vi "dialog.query_string_lua.vi"(5 "LuaVIEW reference":T1) -> (15 "error out":errorcluster)   [LabVIEW 2012]
doc: "Queries for a string by means of a dialog with a string control and OK/Cancel buttons.\nParameters:\nstr:prompt, prompt to display in the dialog titel bar.\n[str:default], default string to set the string control to.\nResults:\nbool:ok, set to true when the query was OKed, false when cancelled.\nstr:string, the entered string."
uses:
  typedefs/t_LuaVIEW Reference.ctl
  subvis/private/LuaVIEW Pull (string).vi
  subvis/private/LuaVIEW Push (boolean).vi
  subvis/private/LuaVIEW Push (string).vi
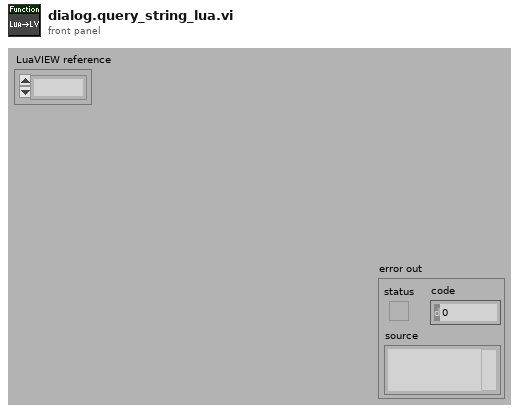
[diagram p1: front panel]
types:
  T1 = typedef "t_LuaVIEW Reference.ctl" = refnum<k1>
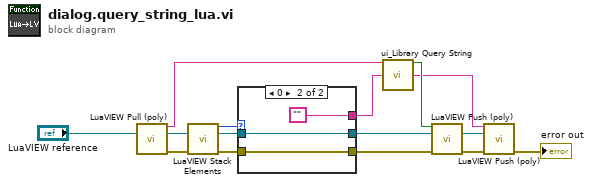
[diagram p0: block diagram]
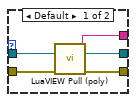
[diagram p2: hidden frame]
diagram:
  n1 = call-poly "LuaVIEW Pull (poly).vi"("LuaVIEW reference in"="LuaVIEW reference") -> ("string"=w7:string, "LuaVIEW reference out"=w13:T1, "error out"=w14:errorcluster)  [unwired: 12 in]
  n2 = call "LuaVIEW Stack Elements.vi"("LuaVIEW reference in"=w13, "error in (no error)"=w14) -> ("elements"=w12:i32, "LuaVIEW reference out"=w10:T1, "error out"=w11:errorcluster)  [unwired: 11 in]
  n3 = case shown="0" w12 {
    tunnel: [w17 ""] -> w6
    tunnel: w11 -> [w20 w23]
    tunnel: w10 -> [w19 w22]
    tunnel: [w18 w23] -> w9
    tunnel: [w16 w22] -> w8
    frame Default {
      n4 = call-poly "LuaVIEW Pull (poly).vi"("LuaVIEW reference in"=w19, "error in (no error)"=w20) -> ("string"=w17:string, "LuaVIEW reference out"=w16:T1, "error out"=w18:errorcluster)  [unwired: 11 in]
    }
    frame 0 {
    }
  }
  n5 = call "ui_Library Query String.vi"("prompt"=w7, "string in (\"\")"=w6) -> ("OKed?"=w5:bool, "string out"=w3:string)  [unwired: 12 in]
  n6 = call-poly "LuaVIEW Push (poly).vi"("boolean"=w5, "LuaVIEW reference in"=w8, "error in (no error)"=w9) -> ("LuaVIEW reference out"=w1:T1, "error out"=w4:errorcluster)  [unwired: 11 in]
  n7 = call-poly "LuaVIEW Push (poly).vi"("string"=w3, "LuaVIEW reference in"=w1, "error in (no error)"=w4) -> ("error out"=→"error out":errorcluster)  [unwired: 11 in, 1 out]
